vi "path_db.vi"(8 "error in":errorcluster) -> (0 "error out":errorcluster, 3 "resulting string":string)   [LabVIEW 2023]
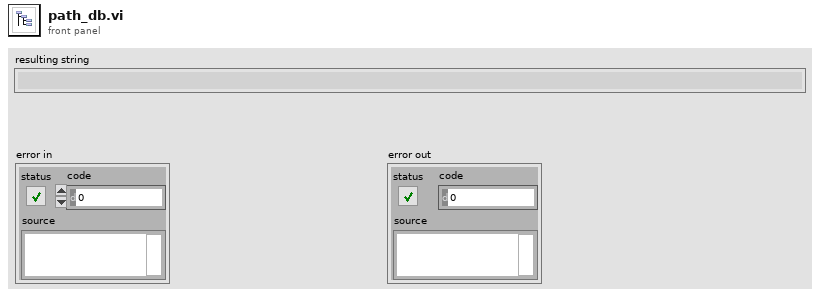
[diagram p1: front panel]
types:
  T1 = enum32{"invalid app kind", "Development System", "Run Time System", "Student Edition", "Embedded LabVIEW", "Evaluation", "Custom"}
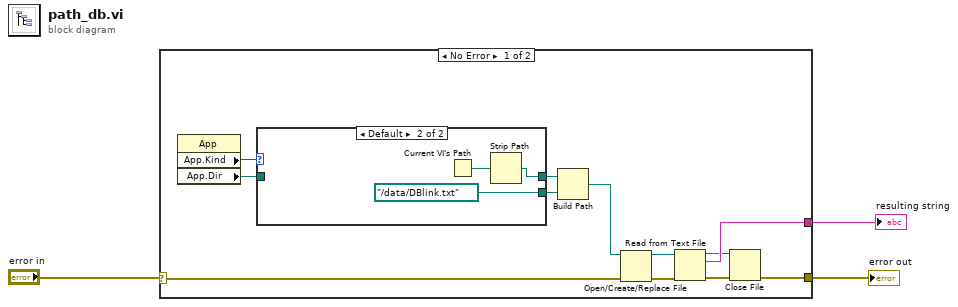
[diagram p0: block diagram]
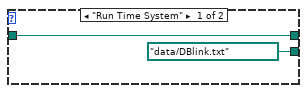
[diagram p2: hidden frame]
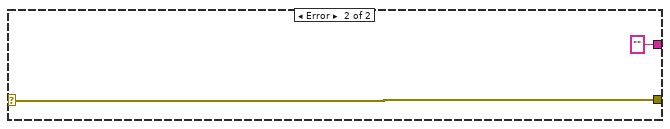
[diagram p3: hidden frame]
diagram:
  n1 = case shown="No Error" "error in" {
    selector: "error in" -> [w4 w22]
    tunnel: [w15 ""] -> w3
    tunnel: [w5 w22] -> w1
    frame No Error {
      n2 = property class="App"() -> ("App.Kind"=w14:T1, "App.Dir"=w13:path)  [unwired: 2 in, 2 out]
      n3 = case shown="Default" w14 {
        tunnel: w13 -> [w17 _]
        tunnel: [path "data/DBlink.txt" ("path") path "../data/DBlink.txt" ("path")] -> w11
        tunnel: [w17 w18] -> w10
        frame "Run Time System" {
        }
        frame Default {
          n4 = Current VI's Path() -> (path=w19:path)
          n5 = Strip Path(path=w19) -> (stripped path=w18:path)  [unwired: 1 out]
        }
      }
      n6 = Build Path(base path=w10, name or relative path=w11) -> (appended path=w12:path)
      n7 = Open/Create/Replace File(file path (use dialog)=w12, error in=w4) -> (refnum out=w7:refnum<file>, error out=w6:errorcluster)  [unwired: 4 in, 1 out]
      n8 = Read from Text File(file (use dialog)=w7, error in=w6) -> (refnum out=w9:refnum<file>, text=w15:string, error out=w8:errorcluster)  [unwired: 2 in, 1 out]
      n9 = Close File(refnum=w9, error in=w8) -> (error out=w5:errorcluster)  [unwired: 1 out]
    }
    frame Error {
    }
  }
  "resulting string" <- w3
  "error out" <- w1
